vi "quadrature watch.vi"(5 "Invert":bool, 7 "Feet Per Second High Gear Full Throttle":dbl, 9 "Feet Per Second Low Gear Full Throttle":dbl, 11 "Throttle state":dbl) -> ()   [LabVIEW 2013]
uses:
  <vilib>/Rock Robotics/SystemInterfaces/DIO/FPGA_DIOChannel.ctl
  <vilib>/Rock Robotics/WPI/Encoder/WPI_EncoderType.ctl
  <vilib>/Rock Robotics/WPI/Counter/WPI_CounterDigitalInputToDigitalSource.vi
panel:
  out "In Range?":bool
  in  "Shifter High":bool
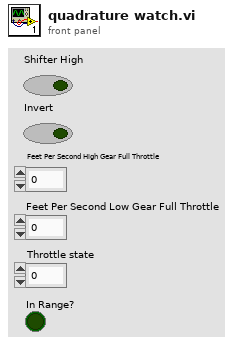
[diagram p1: front panel]
types:
  T1 = typedef "WPI_EncoderType.ctl" = enum16{"1x", "2x", "4x"}
  T2 = typedef "FPGA_DIOChannel.ctl" = enum8{"DIO 1", "DIO 2", "DIO 3", "DIO 4", "DIO 5", "DIO 6", "DIO 7", "DIO 8", "DIO 9", "DIO 10", "DIO 11", "DIO 12", "DIO 13", "DIO 14", "Invalid"}
  T3 = typedef "WPI_DigitalInputDevRef.ctl" = cluster{"DevStatus":errorcluster, "DIO Channel":T2, "Digital Module":T4}
  T4 = typedef "FPGA_TypedefDigitalModule.ctl" = enum16{"Digital Module 1", "Digital Module 2"}
  T5 = typedef "FPGA_CounterEncoderSourceConvertionLVSourceType.ctl" = cluster{"DevStatus":errorcluster, "AnalogTriggerMode?":bool, "DigitalMode":cluster{"Digital Module":T4, "DIO Channel":T6}, "AnalogTriggerMode":cluster{"AnalogTriggerIndex":T7, "OutputType":T8}}
  T6 = typedef "FPGA_DIODigitalSourceChannel.ctl" = enum8{"DIO 1", "DIO 2", "DIO 3", "DIO 4", "DIO 5", "DIO 6", "DIO 7", "DIO 8", "DIO 9", "DIO 10", "DIO 11", "DIO 12", "DIO 13", "DIO 14", "Disabled"}
  T7 = typedef "FPGA_AnalogTriggerIndex.ctl" = enum8{"Trig 0", "Trig 1", "Trig 2", "Trig 3", "Trig 4", "Trig 5", "Trig 6", "Trig 7", "Invalid"}
  T8 = typedef "FPGA_AnalogTriggerOutType.ctl" = enum16{"InWindow", "TriggerState", "Rising", "Falling"}
  T9 = typedef "WPI_EncoderDevRef.ctl" = cluster{"DevStatus":errorcluster, "EncoderIndex":T10, "CounterIndex":T11, "DistancePerCount":dbl, "Decoding Type":T1}
  T10 = typedef "FPGA_EncoderIdx.ctl" = enum8{"Enc 0", "Enc 1", "Enc 2", "Enc 3", "Invalid"}
  T11 = typedef "FPGA_CounterCtrSystemIndex.ctl" = enum8{"Ctr 0", "Ctr 1", "Ctr 2", "Ctr 3", "Ctr 4", "Ctr 5", "Ctr 6", "Ctr 7", "Invalid"}
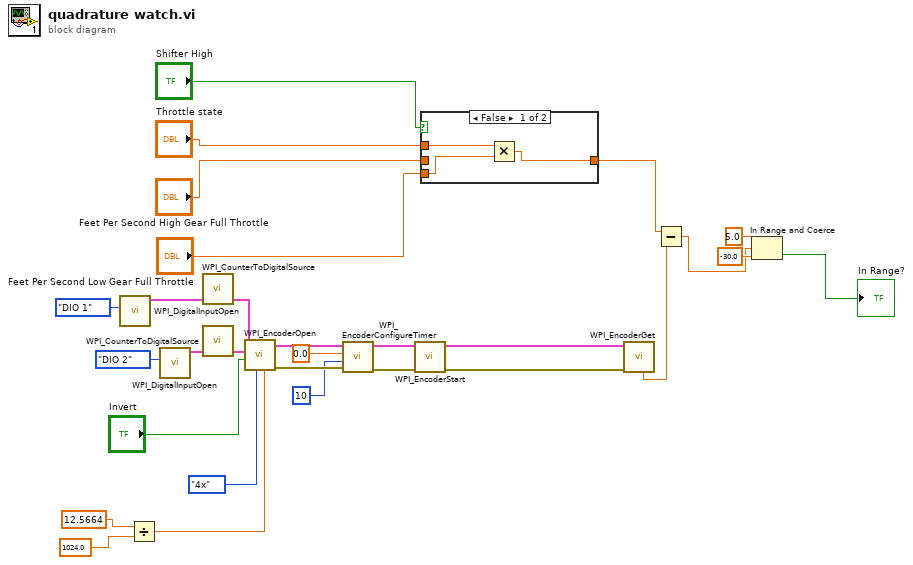
[diagram p0: block diagram]
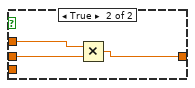
[diagram p2: hidden frame]
diagram:
  n1 = call <vilib>:"WPI_DigitalInputOpen.vi"("DIO Channel"=FPGA_DIOChannel."DIO 1") -> ("DigitalInputDevRef"=w27:T3)  [unwired: 2 in, 8 out]
  n2 = Divide(x=12.5664, y=1024.0) -> (x/y=w15:dbl)
  n3 = call <vilib>:"WPI_DigitalInputOpen.vi"("DIO Channel"=FPGA_DIOChannel."DIO 2") -> ("DigitalInputDevRef"=w28:T3)  [unwired: 2 in, 8 out]
  n4 = call-poly <vilib>:"WPI_CounterToDigitalSource.vi"("DigitalInputDevRef"=w27) -> ("Digital Source"=w26:T5)  [unwired: 6 out]
  n5 = call-poly <vilib>:"WPI_CounterToDigitalSource.vi"("DigitalInputDevRef"=w28) -> ("Digital Source"=w29:T5)  [unwired: 6 out]
  n6 = call <vilib>:"WPI_EncoderOpen.vi"("DistancePerCount"=w15, "Decoding Type"=WPI_EncoderType."4x", "Invert Direction (False)"="Invert", "BSource"=w29, "ASource"=w26) -> ("error out"=w20:errorcluster, "EncoderDevRef"=w21:T9)  [unwired: 3 in, 2 out]
  n7 = call <vilib>:"WPI_EncoderConfigureTimer.vi"("error in (no error)"=w20, "Number Samples to Average"=u8 10, "Minimum Rate"=0.0, "EncoderDevRef"=w21) -> ("error out"=w18:errorcluster, "EncoderDevRef"=w19:T9)  [unwired: 6 in]
  n8 = call <vilib>:"WPI_EncoderStart.vi"("error in (no error)"=w18, "EncoderDevRef"=w19) -> ("error out"=w11:errorcluster, "EncoderDevRef"=w12:T9)  [unwired: 8 in]
  n9 = case shown="False" "Shifter High" {
    tunnel: "Feet Per Second High Gear Full Throttle" -> [_ w35]
    tunnel: "Throttle state" -> [w32 w34]
    tunnel: "Feet Per Second Low Gear Full Throttle" -> [w31 _]
    tunnel: [w30 w33] -> w3
    frame False {
      n10 = Multiply(x=w32, y=w31) -> (x*y=w30:dbl)
    }
    frame True {
      n11 = Multiply(x=w34, y=w35) -> (x*y=w33:dbl)
    }
  }
  n12 = call <vilib>:"WPI_EncoderGet.vi"("error in (no error)"=w11, "EncoderDevRef"=w12) -> ("Rate"=w2:dbl)  [unwired: 4 in, 5 out]
  n13 = Subtract(x=w3, y=w2) -> (x-y=w4:dbl)
  n14 = In Range and Coerce(upper limit=5.0, x=w4, lower limit=-30.0) -> (In Range?=→"In Range?":bool)  [unwired: 1 out]
